vi "IsGUIRunning.vi"(6 "timeout in ms (0)":i32, 8 "Error In":errorcluster, 11 "reference in":refnum<class "UserManager.lvclass">) -> (0 "Error Out":errorcluster, 1 "Running":bool, 3 "reference out":refnum<class "UserManager.lvclass">)   [LabVIEW 2021, in "UserMananger.lvlib" / "UserManager.lvclass"]
uses:
  UserManager.lvclass
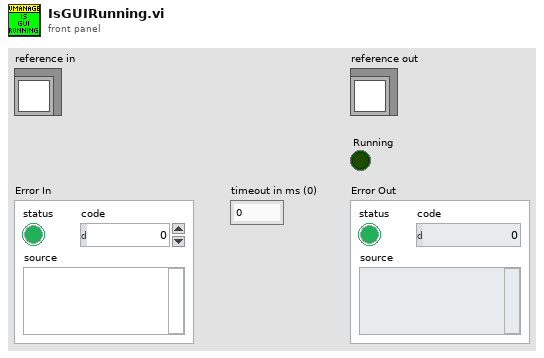
[diagram p1: front panel]
types:
  T1 = typedef "UserMananger.lvlib/UserManager.lvclass/ObjectAttributes.ctl" = cluster{"Interfaces":cluster{"ActivationUpdated":refnum<class "IAuthorizationUpdated.lvclass">}, "Locals":cluster{"MainGUIActive":refnum<queue>, "Evaluations":cluster{"Label":string, "Value":string}[]}, "Persistent":cluster{"Dummy":bool}}
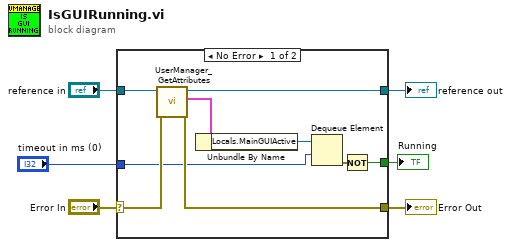
[diagram p0: block diagram]
diagram:
  n1 = case shown="No Error" "Error In" {
    selector: "Error In" -> [w15 w17]
    tunnel: [w8 w17] -> w5
    tunnel: [w12 w16] -> w3
    tunnel: "reference in" -> [w13 w16]
    tunnel: [w11 _] -> w2
    tunnel: "timeout in ms (0)" -> [w7 _]
    frame No Error {
      n2 = call "UserManager_GetAttributes.vi"("error in (no error)"=w15, "reference in"=w13) -> ("error out"=w8:errorcluster, "Data"=w14:T1, "reference out"=w12:refnum<class "UserManager.lvclass">)  [unwired: 6 in, 1 out]
      n3 = Unbundle By Name(w14) -> ("Locals.MainGUIActive"=w10:refnum<queue>)
      n4 = Dequeue Element(queue=w10, timeout in ms (-1)=w7) -> (error out=w9:errorcluster)  [unwired: 1 in, 3 out]
      n5 = Not(x=w9) -> (.not. x?=w11:bool)
    }
    frame Error {
    }
  }
  "Error Out" <- w5
  "reference out" <- w3
  "Running" <- w2
